vi "initial_acquire_sequence.vi"(8 "error in (no error)":errorcluster, 11 "Queue in":refnum<queue>) -> (0 "error out":errorcluster, 3 "queue out":refnum<queue>)   [LabVIEW 2012]
uses:
  typedefs/MicroscopeEvent.ctl
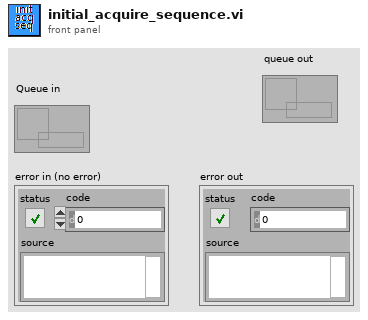
[diagram p1: front panel]
types:
  T1 = typedef "MicroscopeEvent.ctl" = enum16{"M.Wait", "M.RunRotation", "M.Flush", "M.Init", "M.InitStage", "M.InitImageData", "M.ReinitImageData", "M.ReinitImageParams", "M.GetSetParams", "M.InitFastHardware", "M.Pre-Acquire", "M.Acquire", "M.PostAcquire", "M.StopAcquire", "M.SetAcqStatusTrue", "M.SetAcqStatusFalse", "M.ClearImageData", "M.MoveStageDiscrete", "M.MoveStageToTarget1", "M.MoveStageToTarget2", "M.MoveStageToTarget3", "M.OpenShutters", "M.CloseShutters", "M.StartAcquireSequence", "M.ChangeParameters", "M.OpenStokes", "M.OpenPump", "M.RunSW"}
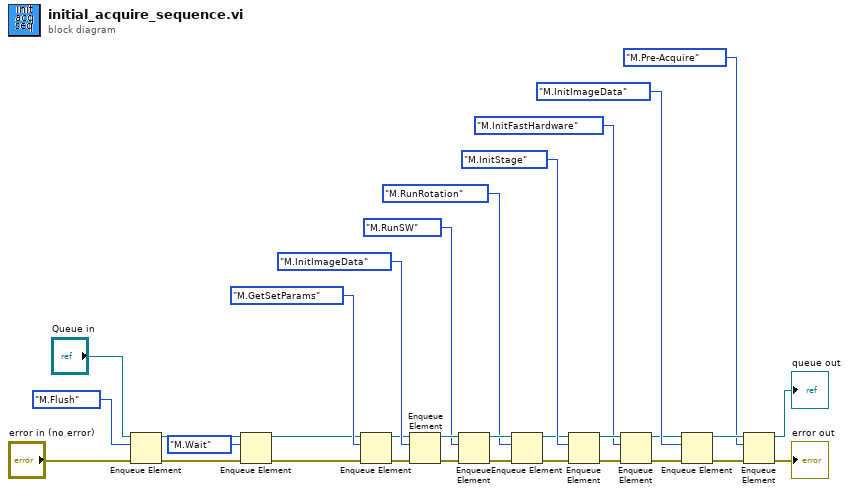
[diagram p0: block diagram]
diagram:
  n1 = Enqueue Element(queue="Queue in", element=MicroscopeEvent."M.Flush", error in (no error)="error in (no error)") -> (queue out=w2:refnum<queue>, error out=w5:errorcluster)  [unwired: 1 in, 1 out]
  n2 = Enqueue Element(queue=w2, element=MicroscopeEvent."M.Wait", error in (no error)=w5) -> (queue out=w3:refnum<queue>, error out=w4:errorcluster)  [unwired: 1 in, 1 out]
  n3 = Enqueue Element(queue=w3, element=MicroscopeEvent."M.GetSetParams", error in (no error)=w4) -> (queue out=w17:refnum<queue>, error out=w9:errorcluster)  [unwired: 1 in, 1 out]
  n4 = Enqueue Element(queue=w17, element=MicroscopeEvent."M.InitImageData" ("t"), error in (no error)=w9) -> (queue out=w19:refnum<queue>, error out=w14:errorcluster)  [unwired: 1 in, 1 out]
  n5 = Enqueue Element(queue=w19, element=MicroscopeEvent."M.RunSW", error in (no error)=w14) -> (queue out=w15:refnum<queue>, error out=w13:errorcluster)  [unwired: 1 in, 1 out]
  n6 = Enqueue Element(queue=w15, element=MicroscopeEvent."M.RunRotation", error in (no error)=w13) -> (queue out=w11:refnum<queue>, error out=w12:errorcluster)  [unwired: 1 in, 1 out]
  n7 = Enqueue Element(queue=w11, element=MicroscopeEvent."M.InitStage", error in (no error)=w12) -> (queue out=w25:refnum<queue>, error out=w26:errorcluster)  [unwired: 1 in, 1 out]
  n8 = Enqueue Element(queue=w25, element=MicroscopeEvent."M.InitFastHardware" ("t"), error in (no error)=w26) -> (queue out=w28:refnum<queue>, error out=w30:errorcluster)  [unwired: 1 in, 1 out]
  n9 = Enqueue Element(queue=w28, element=MicroscopeEvent."M.InitImageData", error in (no error)=w30) -> (queue out=w29:refnum<queue>, error out=w31:errorcluster)  [unwired: 1 in, 1 out]
  n10 = Enqueue Element(queue=w29, element=MicroscopeEvent."M.Pre-Acquire", error in (no error)=w31) -> (queue out=→"queue out":refnum<queue>, error out=→"error out":errorcluster)  [unwired: 1 in, 1 out]
